vi "Monkey operation.vi"(7 "Least Common Multiple":u64, 9 "Value":string, 10 "Operator":string, 11 "Old":u64) -> (3 "New":u64)   [LabVIEW 2021]
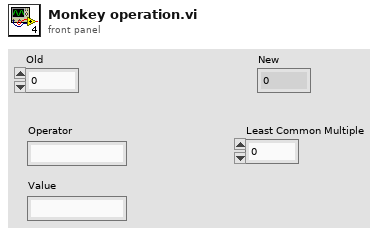
[diagram p1: front panel]
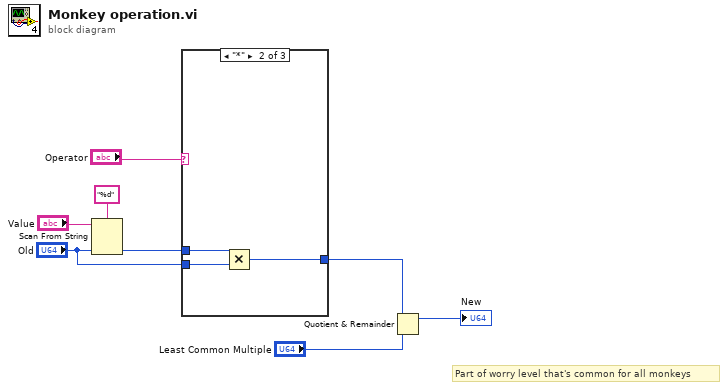
[diagram p0: block diagram]
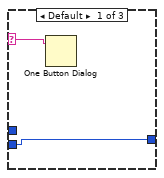
[diagram p2: hidden frame]
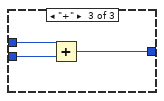
[diagram p3: hidden frame]
diagram:
  # "Part of worry level that's common for all monkeys"
  n1 = Scan From String(format string="%d", input string="Value", default 1="Old") -> (output 1=w5:u64)  [unwired: 2 in, 3 out]
  n2 = case shown="\"*\"" "Operator" {
    selector: "Operator" -> [w10 _ _]
    tunnel: w5 -> [_ w13 w16]
    tunnel: "Old" -> [w9 w12 w15]
    tunnel: [w9 w11 w14] -> w2
    frame Default {
      n3 = One Button Dialog(message=w10) -> ()  [unwired: 1 in, 1 out]
    }
    frame "*" {
      n4 = Multiply(x=w13, y=w12) -> (x*y=w11:u64)
    }
    frame "+" {
      n5 = Add(x=w16, y=w15) -> (x+y=w14:u64)
    }
  }
  n6 = Quotient & Remainder(x=w2, y="Least Common Multiple") -> (x-y*floor(x/y)=→"New":u64)  [unwired: 1 out]
